vi "PH_Beckhoff.get AE Values.vi"(0 "Analog Inputs":T1, 1 "Tags to get":string[](array[string])) -> (2 "Values":dbl[](array[numeric]), 3 "Qualities":bool[](array[boolean]), 4 "Tags not found?":bool[](array[boolean]))   [LabVIEW 2014, in "PH_Beckhoff.lvlib"]
uses:
  PH_Beckhoff.lvlib
  PH_Beckhoff.Analog Inputs.ctl
  PH_Beckhoff.Scaling Type.ctl
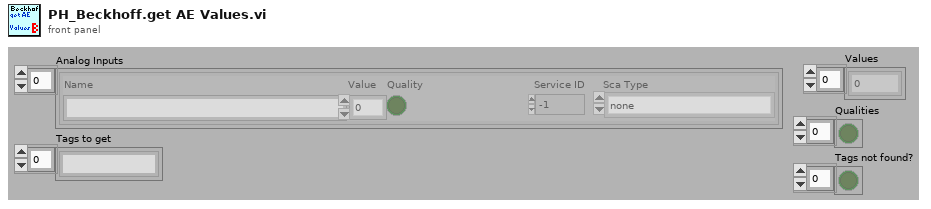
[diagram p1: front panel]
types:
  T1 = typedef "PH_Beckhoff.lvlib/PH_Beckhoff.Analog Inputs.ctl" = cluster{"Name":string, "Value":u32, "Quality":bool, "Service ID":i32, "Sca Type":T2}[]
  T2 = typedef "PH_Beckhoff.lvlib/PH_Beckhoff.Scaling Type.ctl" = enum16{"none", "0 ... 15 Bit -> 0 ... 5", "0 ... 15 Bit -> 0 ... 10", "0 ... 15 Bit -> 0 ... 25", "0 ... 15 Bit -> 4 ... 20", "0 ... 15 Bit -> 0 ... 1", "0 ... 15 Bit -> 0 ... 20000", "0 ... 15 Bit -> 0 ... 24000"}
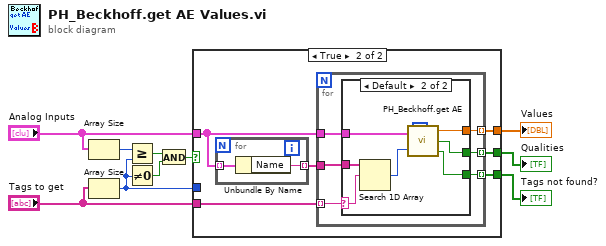
[diagram p0: block diagram]
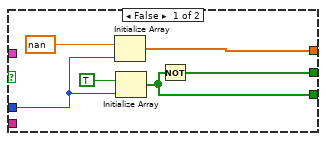
[diagram p2: hidden frame]
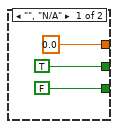
[diagram p3: hidden frame]
diagram:
  n1 = Array Size(array="Analog Inputs") -> (size(s)=w9:i32)
  n2 = Array Size(array="Tags to get") -> (size(s)=w6:i32)
  n3 = Greater Or Equal?(x=w9, y=w6) -> (x >= y?=w3:bool)
  n4 = Not Equal To 0?(x=w6) -> (x != 0?=w4:bool)
  n5 = And(x=w3, y=w4) -> (x .and. y?=w5:bool)
  n6 = case shown="True" w5 {
    tunnel: [w15 w19] -> w2
    tunnel: [w11 w17] -> w10
    tunnel: [w14 w18] -> w1
    tunnel: "Tags to get" -> [_ w20]
    tunnel: "Analog Inputs" -> [_ w22]
    tunnel: w6 -> [w13 _]
    frame False {
      n7 = Initialize Array(nan, w13) -> (w11:dbl[])
      n8 = Initialize Array(TRUE, w13) -> (w15:bool[])
      n9 = Not(x=w15) -> (.not. x?=w14:bool[])
    }
    frame True {
      n10 = for {
        tunnel: w22 -> [w40] mode=indexing
        tunnel: [w39] -> w21 mode=indexing
        n11 = Unbundle By Name(w40) -> ("Name"=w39:string)
      }
      n12 = for {
        tunnel: w22 -> [w28]
        tunnel: [w27] -> w17 mode=indexing
        tunnel: [w26] -> w18 mode=indexing
        tunnel: [w25] -> w19 mode=indexing
        tunnel: w21 -> [w24]
        tunnel: w20 -> [w23] mode=indexing
        n13 = case shown="Default" w23 {
          selector: w23 -> [_ w32]
          tunnel: w28 -> [_ w38]
          tunnel: [0.0 ("DIM value") w37] -> w27
          tunnel: [TRUE ("Quality") w36] -> w26
          tunnel: [FALSE w34] -> w25
          tunnel: w24 -> [_ w33]
          frame "", "N/A" {
          }
          frame Default {
            n14 = Search 1D Array(1D array=w33, element=w32) -> (index of element=w35:i32)  [unwired: 1 in]
            n15 = call "PH_Beckhoff.get AE.vi"("Analog Inputs"=w38, "index of element"=w35) -> ("DIM value"=w37:dbl, "Quality"=w36:bool, "Tag not found"=w34:bool)
          }
        }
      }
    }
  }
  "Tags not found?" <- w2
  "Qualities" <- w1
  "Values" <- w10
